vi "transmitter.vi"() -> ()   [LabVIEW 2013]
uses:
  <instrlib>/niUSRP/niUSRP Write Tx Data (CDB).vi
panel:
  out "error out":errorcluster
  out "coerced gain":dbl format="%#_6f"
  out "coerced carrier frequency":dbl=100000.0 format="%#_6p"
  out "coerced IQ rate":dbl=100000.0 format="%#_6p"
  in  "stop":bool
  in  "active antenna":string
  in  "gain":dbl format="%#_6f"
  in  "carrier frequency":dbl=100000.0 format="%#_6p"
  in  "IQ rate":dbl=100000.0 format="%#_6p"
  in  "waveform size":i32
  in  "device names":refnum<k15>
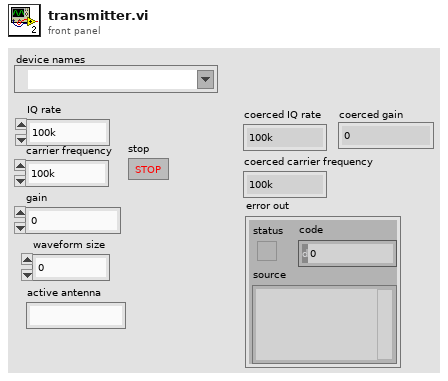
[diagram p1: front panel]
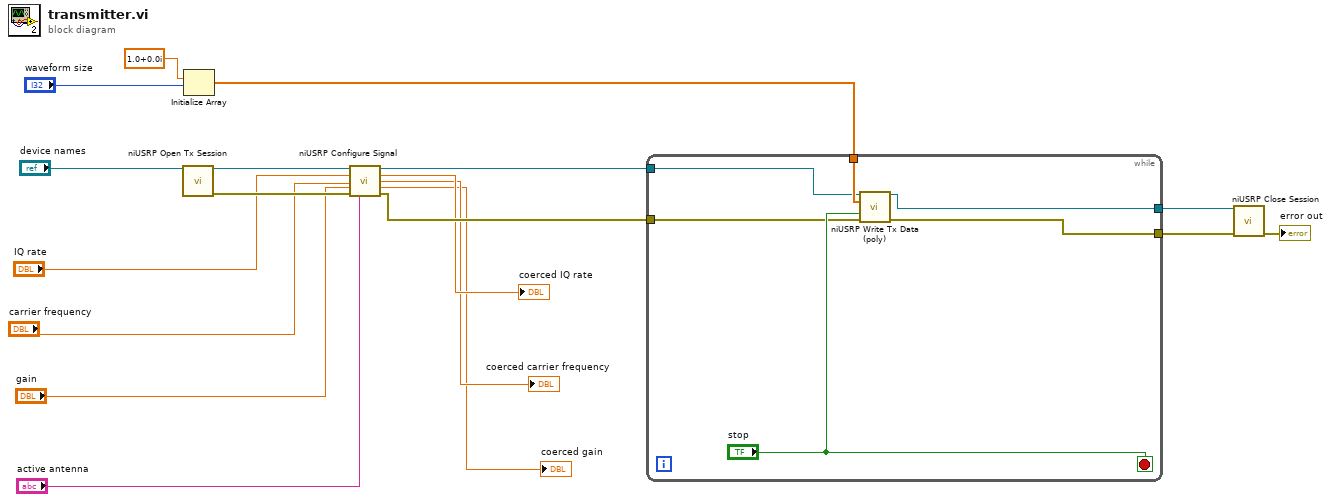
[diagram p0: block diagram]
diagram:
  n1 = call <instrlib>:"niUSRP Open Tx Session.vi"("device names"="device names") -> ("session handle out"=w15:refnum<k15>, "error out"=w14:errorcluster)  [unwired: 13 in]
  n2 = Initialize Array(cdb 1.0+0.0i, "waveform size") -> (w9:cdb[])
  n3 = call <instrlib>:"niUSRP Configure Signal.vi"("session handle"=w15, "IQ rate"="IQ rate", "carrier frequency"="carrier frequency", "gain"="gain", "error in (no error)"=w14, "active antenna"="active antenna") -> ("session handle out"=w8:refnum<k15>, "coerced IQ rate"=→"coerced IQ rate":dbl, "coerced carrier frequency"=→"coerced carrier frequency":dbl, "coerced gain"=→"coerced gain":dbl, "error out"=w7:errorcluster)  [unwired: 5 in]
  n4 = while {
    tunnel: w9 -> [w23]
    tunnel: w8 -> [w22]
    tunnel: w7 -> [w21]
    tunnel: [w20] -> w3
    tunnel: [w19] -> w2
    stop <- "stop" stop-if-true
    n5 = call-poly <instrlib>:"niUSRP Write Tx Data (poly).vi"("session handle"=w22, "data"=w23, "end of data?"="stop", "error in (no error)"=w21) -> ("session handle out"=w20:refnum<k15>, "error out"=w19:errorcluster)  [unwired: 10 in]
  }
  n6 = call <instrlib>:"niUSRP Close Session.vi"("session handle"=w3, "error in (no error)"=w2) -> ("error out"=→"error out":errorcluster)  [unwired: 13 in]
